vi "Read Packet Buffer.vi"(0 "data fifo":refnum<k21>, 1 "reset":bool, 5 "sizes fifo":refnum<k21>, 12 "ready for output":bool) -> (3 "in reset":bool, 4 "serialized data":u8[](array[numeric]), 6 "valid bytes":fxp<+,4,4>, 8 "empty":bool, 10 "output valid":bool)   [LabVIEW 2020, in "GettingStarted_Acq_Tap_148X_FPGA.lvlib"]
uses:
  <instrlib>/FlexRIO/CSI-2/v2/FPGA/Types/Read Packet Buffer State.ctl
  <instrlib>/FlexRIO/CSI-2/v2/FPGA/Types/Read Packet Buffer State Data.ctl
  <vilib>/rvi/DataTransferAndStorage/Container/Common/niFpgaContainerExecOnDevCompGetState.vi
  <vilib>/rvi/Emulation/niFpgaEmulationIsFPGAContextNoSignature.vi
  <vilib>/rvi/Emulation/niFpgaSctlEmulationGetInTimedLoop.vi
  <vilib>/rvi/errors/niFpgaSetErrorForExecOnDevCompSimple.vi
  <vilib>/rvi/eio/common/nirviEmuReportErrorAndStop.vi
  <vilib>/rvi/DataTransferAndStorage/Container/Common/niFpgaContainerGetUniqueNameForEmu.vi
  <vilib>/rvi/FIFO/Fifo_Resource/nirvififoEmulationSetSize.vi
  <vilib>/rvi/FIFO/Fifo_Resource/nirviFifoEmulationQueueMgr.vi
  <instcachedir>/0/nirviFifoEmulationQueueMgr_E5CAEC123FF24DC58D834DCA3CDAA9B5.lvgen/nirviFifoEmulationQueueMgr_E5CAEC123FF24DC58D834DCA3CDAA9B5_012.vi
  <vilib>/rvi/FIFO/Fifo_Resource/nirvififoEmulationDetermineInputValidOut.vi
  <vilib>/rvi/FIFO/Fifo_Resource/nirvififoEmulationCreateLock.vi
  <vilib>/rvi/Emulation/niFpgaProcessEmulError.vi
  <vilib>/rvi/FIFO/Fifo_Resource/nirvififoEmulationObtainLock.vi
  <vilib>/rvi/FIFO/Fifo_Resource/nirvififoEmulationReleaseLock.vi
  <vilib>/rvi/occurrence/nirviWaitOnOccurrenceBase.vi
  <vilib>/rvi/errors/nirviReportUnexpectedCaseInternalError.vi
  <vilib>/rvi/errors/nirviReportUnexpectedCaseInternalError (U32).vi
  <vilib>/Utility/error.llb/Clear Errors.vi
  <vilib>/rvi/interface/RandomDataEmulation/niFpgaRandomDataHandleErrors.vi
  <instcachedir>/0/nirviFifoEmulationQueueMgr_E5CAEC123FF24DC58D834DCA3CDAA9B5.lvgen/nirviFifoEmulationQueueMgr_E5CAEC123FF24DC58D834DCA3CDAA9B5_000.vi
  <instrlib>/_niInstr/Data Formatting/v1/FPGA/Private/Convert/Boolean Array to U8 Array.vi
  035627ac-b731-4cad-8467-faa712293712.vi
  <vilib>/rvi/DataTransferAndStorage/Container/XNode/niFpgaContainer.xnode
  <vilib>/rvi/FIFO/Fifo_Resource/niFpgaFifoEmulationRefIn.vi
  GettingStarted_Acq_Tap_148X_FPGA.lvlib
  <instrlib>/_niInstr/Data Formatting/v1/FPGA/niInstr Data Formatting v1 FPGA.lvlib
  <instrlib>/FlexRIO/CSI-2/v2/FPGA/NI CSI-2 API FPGA v2.lvlib
  <instrlib>/_niInstr/Basic Elements/v1/FPGA/niInstr Basic Elements v1 FPGA.lvlib
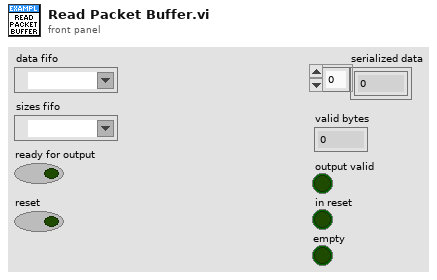
[diagram p1: front panel]
types:
  T1 = typedef "NI CSI-2 API FPGA v2.lvlib/Read Packet Buffer State.ctl" = enum8{"read timestamp", "read size and header", "read payload"}
  T2 = typedef "NI CSI-2 API FPGA v2.lvlib/Read Packet Buffer State Data.ctl" = cluster{"state":T1, "bytes remaining":fxp<+,17,17>}
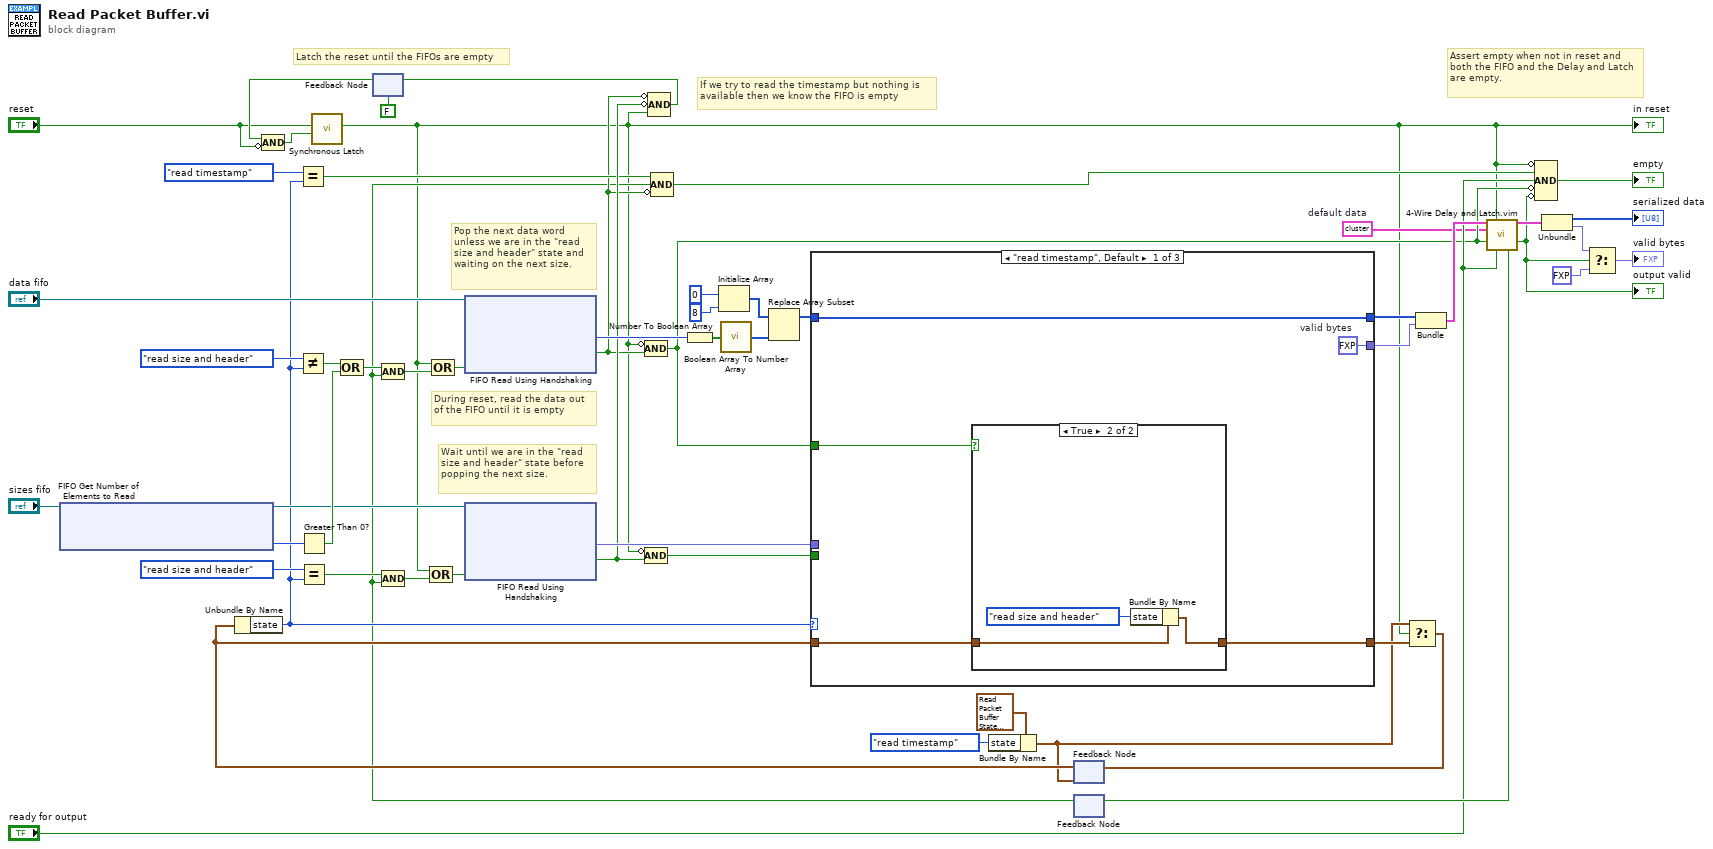
[diagram p0: block diagram]
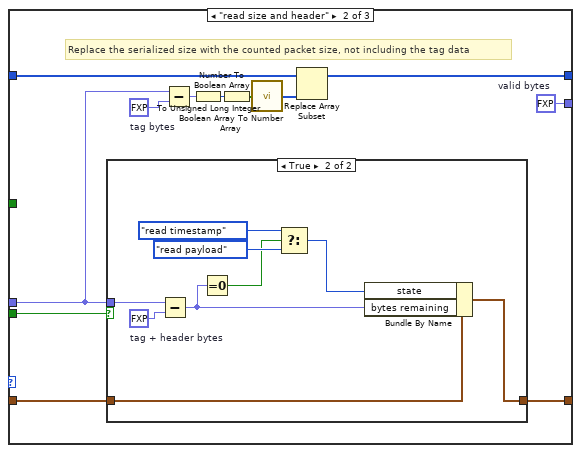
[diagram p3: hidden frame]
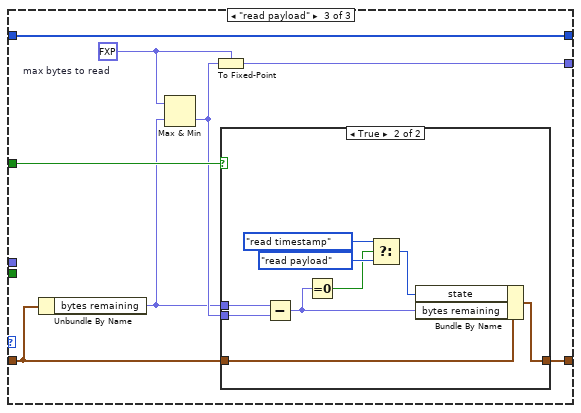
[diagram p5: hidden frame]
diagram:
  w6 = cluster{u8[], "max bytes to read":fxp<+,4,4>} {[0, 0, 0, 0, 0, 0, 0, 0], "max bytes to read"=0.0}  # default data
  # "Assert empty when not in reset and both the FIFO and the Delay and Latch are empty."
  # "If we try to read the timestamp but nothing is available then we know the FIFO is empty"
  # "Latch the reset until the FIFOs are empty"
  # "During reset, read the data out of the FIFO until it is empty"
  # "Pop the next data word unless we are in the \"read size and header\" state and waiting on the next size."
  # "Wait until we are in the \"read size and header\" state before popping the next size."
  n1 = xnode ("FIFO Get Number of Elements to Read")("FIFO In"="sizes fifo") -> ("Number of Elements to Read"=w35:u32, "FIFO Out"=w39:refnum<k21>)
  n2 = Greater Than 0?(x=w35) -> (x > 0?=w45:bool)
  n3 = feedback #1(FALSE) -> (w4:bool)
  n4 = Compound Arithmetic op=AND(w4, invert "reset") -> (w5:bool)
  n5 = call <instrlib>:"Synchronous Latch.vi"("clear"=w5, "set"="reset") -> ("out"=w1:bool)  [unwired: 9 in]
  "in reset" <- w1
  n6 = Initialize Array(u8 0 ("element"), 8 ("dimension size")) -> (w29:u8[])
  n7 = Bundle By Name(cluster=T2 {"state"=enum."read timestamp", "bytes remaining"=0.0}, "state"=Read_Packet_Buffer_State."read timestamp") -> (w2:T2)
  n8 = feedback #2(w2) -> (w55:T2)
  n9 = Unbundle By Name(w55) -> ("state"=w16:T1)
  n10 = Equal?(x=Read_Packet_Buffer_State."read timestamp", y=w16) -> (x = y?=w14:bool)
  n11 = Not Equal?(x=Read_Packet_Buffer_State."read size and header", y=w16) -> (x != y?=w43:bool)
  n12 = Equal?(x=Read_Packet_Buffer_State."read size and header", y=w16) -> (x = y?=w28:bool)
  n13 = Compound Arithmetic op=OR(w43, w45) -> (w46:bool)
  n14 = feedback #3() -> (w12:bool)  [unwired: 1 in]
  n15 = Compound Arithmetic op=AND(w46, w12) -> (w25:bool)
  n16 = Compound Arithmetic op=AND(w28, w12) -> (w27:bool)
  n17 = Compound Arithmetic op=OR(w1, w27) -> (w26:bool)
  n18 = Compound Arithmetic op=OR(w1, w25) -> (w24:bool)
  n19 = xnode ("FIFO Read Using Handshaking")("Ready for Output"=w24, "FIFO In"="data fifo") -> ("Element"=w41:u64, "Output Valid"=w13:bool)  [unwired: 1 out]
  n20 = xnode ("FIFO Read Using Handshaking")("Ready for Output"=w26, "FIFO In"=w39) -> ("Element"=w47:fxp<+,17,17>, "Output Valid"=w22:bool)  [unwired: 1 out]
  n21 = Compound Arithmetic op=AND(invert w1, w13) -> (w7:bool)
  n22 = Compound Arithmetic op=AND(invert w1, w22) -> (w34:bool)
  n23 = Compound Arithmetic op=AND(invert w13, invert w22, w1) -> (w37:bool)
  n24 = feedback-in #1(w37) -> ()
  n25 = Compound Arithmetic op=AND(w14, w12, invert w13) -> (w11:bool)
  n26 = Number To Boolean Array(number=w41) -> (Boolean array=w42:bool[])
  n27 = call-poly <instrlib>:"Boolean Array To Number Array.vi"("data in"=w42) -> ("data out"=w33:u8[])  [unwired: 14 in]
  n28 = Replace Array Subset(array=w29, new element=w33) -> (w32:u8[])  [unwired: 1 in]
  n29 = case shown="\"read timestamp\", Default" w16 {
    tunnel: w32 -> [w61 w77 w95]
    tunnel: [w61 w76 w95] -> w48
    tunnel: w34 -> [_ w67 _]
    tunnel: [w57 w66 w88] -> w49
    tunnel: w55 -> [w60 w75 w93]
    tunnel: [w59 w74 w94] -> w53
    tunnel: w47 -> [_ w73 _]
    tunnel: w7 -> [w58 _ w92]
    frame "read timestamp", Default {
      w57 = fxp<+,4,4> 8.0  # valid bytes
      n30 = case shown="True" w58 {
        tunnel: w60 -> [w62 w65]
        tunnel: [w62 w64] -> w59
        frame False {
        }
        frame True {
          n31 = Bundle By Name(cluster=w65, "state"=Read_Packet_Buffer_State."read size and header") -> (w64:T2)
        }
      }
    }
    frame "read size and header" {
      w66 = fxp<+,4,4> 8.0  # valid bytes
      w69 = fxp<+,17,17> 12.0  # tag bytes
      # "Replace the serialized size with the counted packet size, not including the tag data"
      n32 = case shown="True" w67 {
        tunnel: w75 -> [w78 w87]
        tunnel: [w78 w86] -> w74
        tunnel: w73 -> [_ w85]
        frame False {
        }
        frame True {
          w84 = fxp<+,17,17> 16.0  # tag + header bytes
          n33 = Subtract(x=w85, y=w84) -> (x-y=w81:fxp<+,17,17>)
          n34 = Equal To 0?(x=w81) -> (x = 0?=w79:bool)
          n35 = Select(t=Read_Packet_Buffer_State."read timestamp", s=w79, f=Read_Packet_Buffer_State."read payload") -> (s? t:f=w80:T1)
          n36 = Bundle By Name(cluster=w87, "state"=w80, "bytes remaining"=w81) -> (w86:T2)
        }
      }
      n37 = Subtract(x=w73, y=w69) -> (x-y=w68:fxp<+,17,17>)
      n38 = To Unsigned Long Integer(number=w68) -> (unsigned 32bit integer=w72:u32)
      n39 = Number To Boolean Array(number=w72) -> (Boolean array=w71:bool[])
      n40 = call-poly <instrlib>:"Boolean Array To Number Array.vi"("data in"=w71) -> ("data out"=w70:u8[])  [unwired: 14 in]
      n41 = Replace Array Subset(array=w77, new element=w70) -> (w76:u8[])  [unwired: 1 in]
    }
    frame "read payload" {
      w90 = fxp<+,4,4> 8.0  # max bytes to read
      n42 = Unbundle By Name(w93) -> ("bytes remaining"=w89:fxp<+,17,17>)
      n43 = Max & Min(x=w90, y=w89) -> (min(x,y)=w91:fxp<+,17,17>)  [unwired: 1 out]
      n44 = To Fixed-Point(fixed-point type=w90, number=w91) -> (fixed-point=w88:fxp<+,4,4>)
      n45 = case shown="True" w92 {
        tunnel: [w96 w100] -> w94
        tunnel: w93 -> [w96 w99]
        tunnel: w91 -> [_ w98]
        tunnel: w89 -> [_ w97]
        frame False {
        }
        frame True {
          n46 = Subtract(x=w97, y=w98) -> (x-y=w103:fxp<+,17,17>)
          n47 = Equal To 0?(x=w103) -> (x = 0?=w101:bool)
          n48 = Select(t=Read_Packet_Buffer_State."read timestamp", s=w101, f=Read_Packet_Buffer_State."read payload") -> (s? t:f=w102:T1)
          n49 = Bundle By Name(cluster=w99, "state"=w102, "bytes remaining"=w103) -> (w100:T2)
        }
      }
    }
  }
  n50 = Select(t=w2, s=w1, f=w53) -> (s? t:f=w54:T2)
  n51 = feedback-in #2(w54) -> ()
  n52 = Bundle(w48, "max bytes to read"=w49) -> (w50:cluster{u8[], "max bytes to read":fxp<+,4,4>})  [unwired: 1 in]
  n53 = call "4-Wire Delay and Latch.vim"("data in"=w50, "reset"=w1, "default data"=w6, "input valid"=w7, "ready for output"="ready for output") -> ("data out"=w51:cluster{u8[], "max bytes to read":fxp<+,4,4>}, "output valid"=w8:bool, "ready for input"=w56:bool)  [unwired: 8 in]
  "output valid" <- w8
  n54 = feedback-in #3(w56) -> ()
  n55 = Compound Arithmetic op=AND(invert w1, w11, "ready for output", invert w7, invert w8) -> (→"empty":bool)
  n56 = Unbundle(w51) -> (→"serialized data":u8[], "max bytes to read"=w20:fxp<+,4,4>)
  n57 = Select(t=w20, s=w8, f=fxp<+,4,4> 0.0) -> (s? t:f=→"valid bytes":fxp<+,4,4>)
